vi "serialPorts.vi"(11 "Python version":string) -> (0 "error out":errorcluster, 1 "ports":string[](array[string]), 2 "appended path":path, 3 "Refnum out":refnum<k35>)   [LabVIEW 2019]
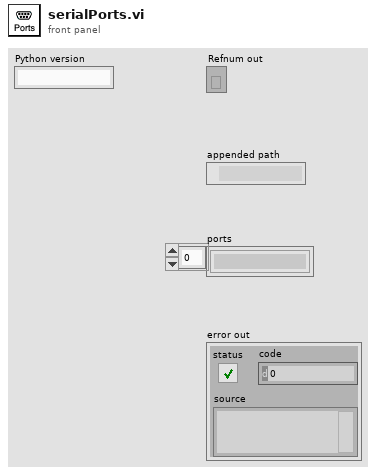
[diagram p1: front panel]
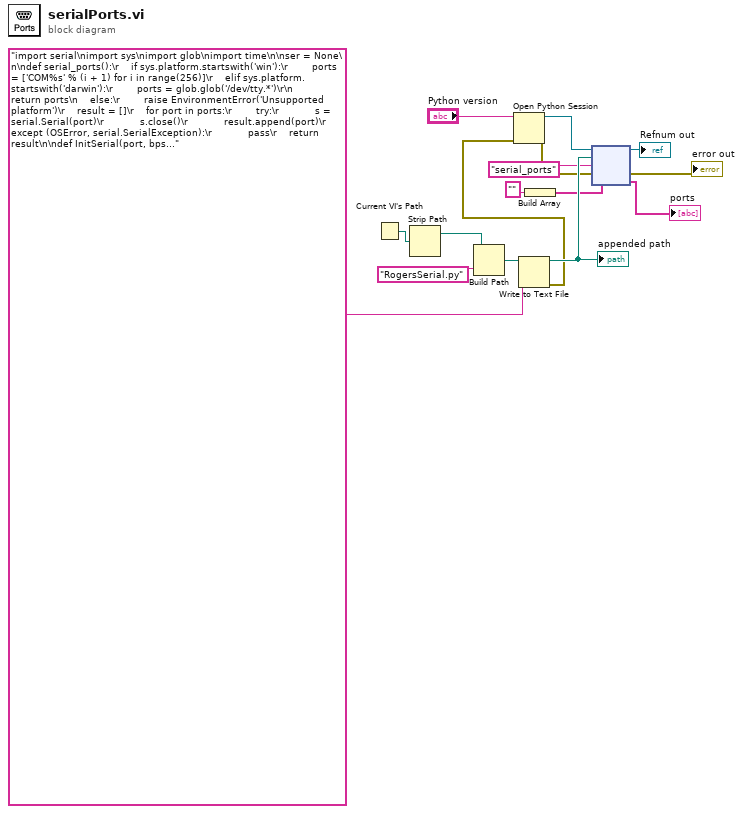
[diagram p0: block diagram]
diagram:
  n1 = Current VI's Path() -> (path=w9:path)
  n2 = Strip Path(path=w9) -> (stripped path=w10:path)  [unwired: 1 out]
  n3 = Build Path(base path=w10, name or relative path="RogersSerial.py") -> (appended path=w15:path)
  "appended path" <- w15
  n4 = Write to Text File(file (use dialog)=w15, text="import serial\nimport sys\nimport glob\nimport time\n\nser = None\n\ndef serial_ports():\r    if sys.platform.startswith('win'):\r        ports = ['COM%s' % (i + 1) for i in range(256)]\r    elif sys.platform.startswith('darwin'):\r        ports = glob.glob('/dev/tty.*')\r\n        return ports\n    else:\r        raise EnvironmentError('Unsupported platform')\r    result = []\r    for port in ports:\r        try:\r            s = serial.Serial(port)\r            s.close()\r            result.append(port)\r        except (OSError, serial.SerialException):\r            pass\r    return result\n\ndef InitSerial(port, bps = 9600, to = 0):\n    global ser\n    ser = serial.Serial(port, bps, timeout = to)  # open serial port\n    return (ser.name)\n\ndef CloseSerial():\n    global ser\n    ser.close()\n    return('done')\n\ndef WriteSerial(string):\n    global ser\n    return(ser.write(string.encode()))    # write a string\n\ndef ScriptSerial(string):\n    global ser\n    reply = ''\n    lines = string.split('\\n')\n    for line in lines:\n        ser.write(line.encode())\n        time.sleep(1)\n        reply += ReadSerial() + '\\n'\n    return reply \n\ndef ReadSerial():\n    global ser\n    reply = ''\n    if ser.in_waiting:\n        reply = ser.read(ser.in_waiting).decode()\n    return(reply)\n") -> (error out=w2:errorcluster)  [unwired: 2 in, 2 out]
  n5 = Open Python Session(python version="Python version", 3:w2) -> (session out=w14:refnum<k35>, error out=w1:errorcluster)  [unwired: 1 in]
  n6 = Build Array("" ("function name")) -> (w6:string[])
  n7 = node(w14, w15, "serial_ports" ("function name"), w1, w6) -> (→"Refnum out":refnum<k35>, →"error out":errorcluster, →"ports":string[])  [unwired: 2 out]
